vi "Create UNSUBSCRIBE Packet.vi"(5 "UNSUBSCRIBE in":refnum<class "UNSUBSCRIBE.lvclass">, 8 "error in (no error)":errorcluster, 9 "Packet ID":u16 format="%04x", 11 "Topic Subscriptions":string[](array[string])) -> (0 "error out":errorcluster, 3 "UNSUBSCRIBE out":refnum<class "UNSUBSCRIBE.lvclass">)   [LabVIEW 2013, in "UNSUBSCRIBE.lvclass"]
uses:
  UNSUBSCRIBE.lvclass
  ControlPacket/ControlPacket.lvclass/ControlPacket.ctl
  ControlPacket/ControlPacket.lvclass
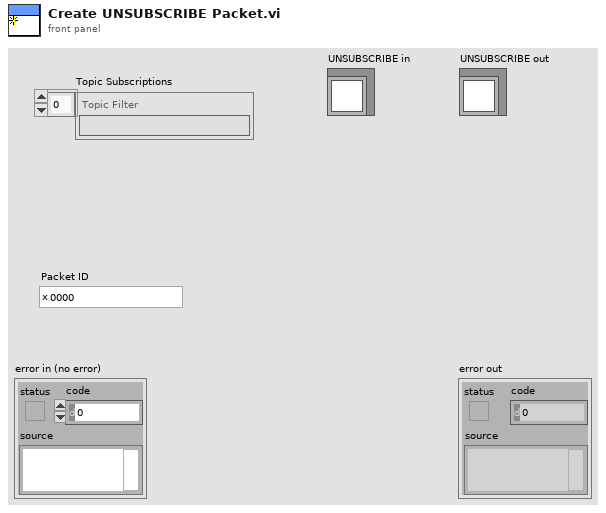
[diagram p1: front panel]
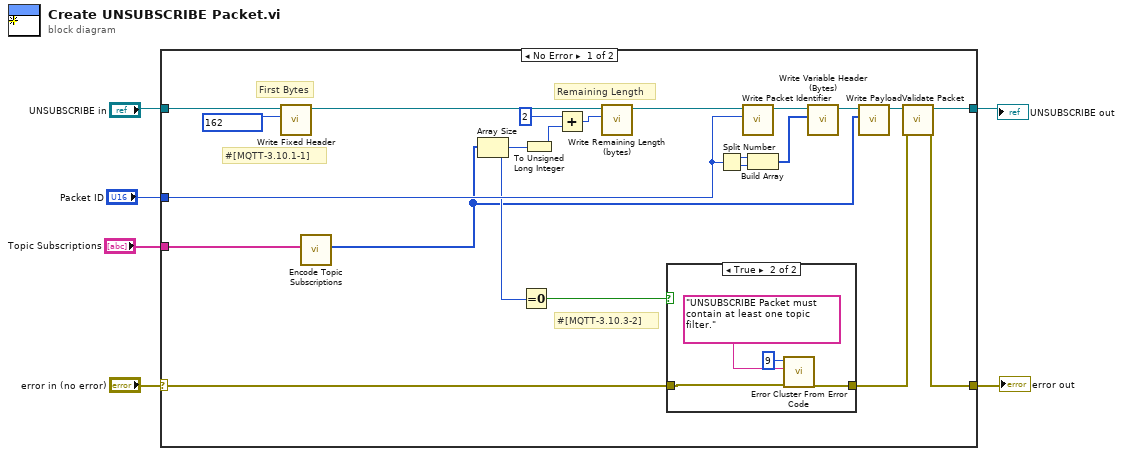
[diagram p0: block diagram]
diagram:
  n1 = case shown="No Error" "error in (no error)" {
    selector: "error in (no error)" -> [w14 w35]
    tunnel: [w9 w35] -> w2
    tunnel: [w11 w34] -> w1
    tunnel: "UNSUBSCRIBE in" -> [w28 w34]
    tunnel: "Packet ID" -> [w20 _]
    tunnel: "Topic Subscriptions" -> [w8 _]
    frame No Error {
      # "#[MQTT-3.10.3-2]"
      # "#[MQTT-3.10.1-1]"
      # "Remaining Length"
      # "First Bytes"
      n2 = call "Write Fixed Header.vi"("Fixed Header"=u8 162, "ControlPacket in"=w28) -> ("ControlPacket out"=w27:refnum<class "UNSUBSCRIBE.lvclass">)  [unwired: 9 in]
      n3 = call "Encode Topic Subscriptions.vi"("Topic Subscriptions"=w8) -> ("Length-Prefixed Field"=w7:u8[])  [unwired: 10 in]
      n4 = Array Size(array=w7) -> (size(s)=w15:i32)
      n5 = Equal To 0?(x=w15) -> (x = 0?=w13:bool)
      n6 = To Unsigned Long Integer(number=w15) -> (unsigned 32bit integer=w16:u32)
      n7 = Add(x=u32 2 ("Remaining Length (bytes)"), y=w16) -> (x+y=w18:u32)
      n8 = call "Write Remaining Length (bytes).vi"("Remaining Length (bytes)"=w18, "ControlPacket in"=w27) -> ("ControlPacket out"=w23:refnum<class "UNSUBSCRIBE.lvclass">)  [unwired: 9 in]
      n9 = case shown="True" w13 {
        tunnel: w14 -> [w29 w32]
        tunnel: [w29 w33] -> w10
        frame False {
        }
        frame True {
          n10 = call <vilib>:"Error Cluster From Error Code.vi"("error in (no error)"=w32, "error message (\"\")"="UNSUBSCRIBE Packet must contain at least one topic filter.", "error code (0)"=9) -> ("error out"=w33:errorcluster)  [unwired: 6 in]
        }
      }
      n11 = Split Number(x=w20) -> (hi(x)=w26:u8, lo(x)=w25:u8)
      n12 = call "Write Packet Identifier.vi"("Packet Identifier"=w20, "ControlPacket in"=w23) -> ("ControlPacket out"=w22:refnum<class "UNSUBSCRIBE.lvclass">)  [unwired: 9 in]
      n13 = Build Array(w26, w25) -> (w24:u8[])
      n14 = call "Write Variable Header (Bytes).vi"("Variable Header (Bytes)"=w24, "ControlPacket in"=w22) -> ("ControlPacket out"=w17:refnum<class "UNSUBSCRIBE.lvclass">)  [unwired: 9 in]
      n15 = call "Write Payload.vi"("Payload"=w7, "ControlPacket in"=w17) -> ("ControlPacket out"=w12:refnum<class "UNSUBSCRIBE.lvclass">)  [unwired: 9 in]
      n16 = call "Validate Packet.vi"("error in (no error)"=w10, "ControlPacket in"=w12) -> ("error out"=w9:errorcluster, "ControlPacket out"=w11:refnum<class "UNSUBSCRIBE.lvclass">)  [unwired: 8 in]
    }
    frame Error {
    }
  }
  "error out" <- w2
  "UNSUBSCRIBE out" <- w1
